vi "punto3_readfrom.vi"() -> ()   [LabVIEW 2024]
uses:
  <vilib>/express/express analysis/Spectral/Block/exnSpectralBlock spectral measurements peak poly.vi
  <vilib>/express/express analysis/Spectral/Block/exnSpectralBlock spectral measurements peak DDT.vi
  <vilib>/express/express analysis/Spectral/Block/exnSpectralBlock spectral measurements power poly.vi
  <vilib>/express/express analysis/Spectral/Block/exnSpectralBlock spectral measurements power DDT.vi
  <vilib>/express/express analysis/Spectral/XNode/ExpressSpectralMeasurementsBlockNode.xnode
panel:
  out "SINAD":dbl
  out "THD":dbl
  out "NOISE":dynamicdata(graph)
  out "SNR":dbl
  out "dt":dbl
  out "Y":dbl[](array[numeric])
  out "SIGNAL":dynamicdata(graph)
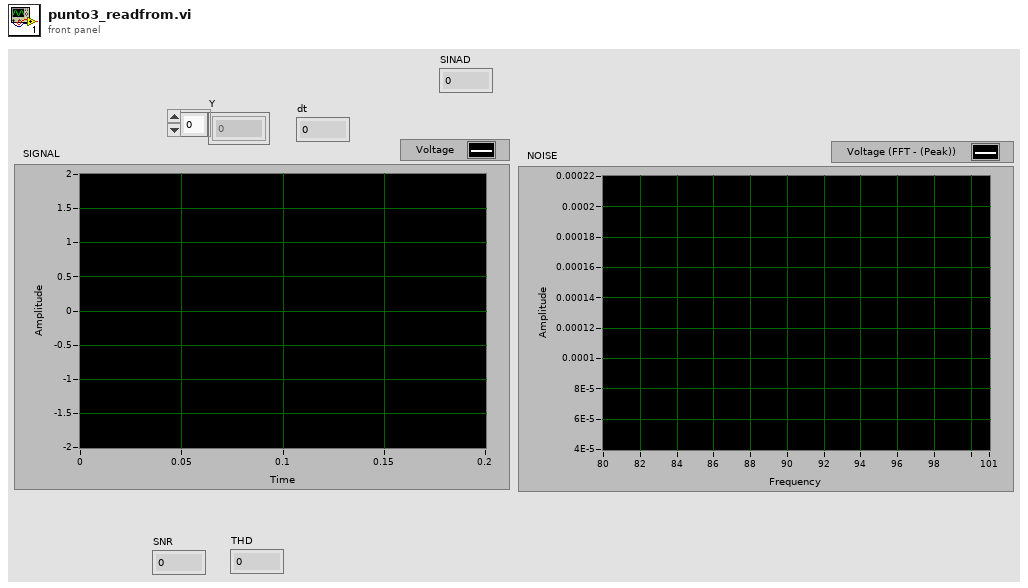
[diagram p1: front panel]
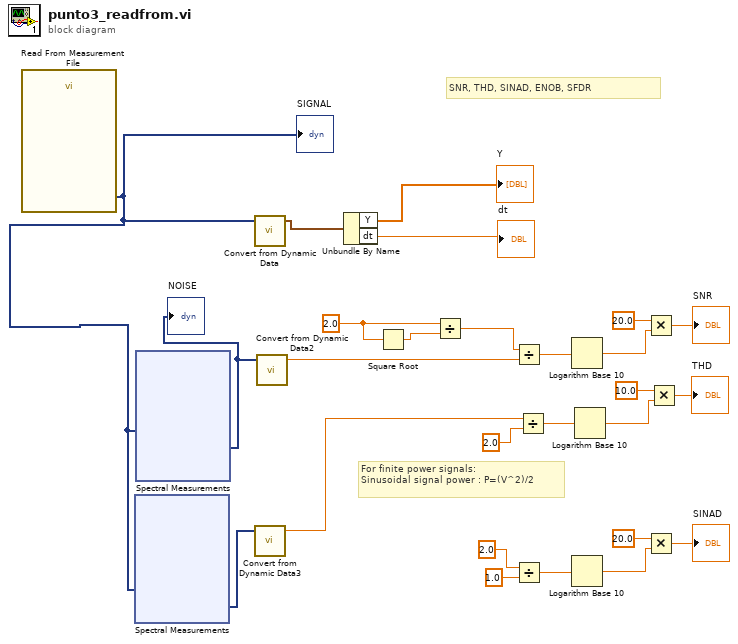
[diagram p0: block diagram]
diagram:
  w18 = 2.0 ("x")
  # "For finite power signals:\nSinusoidal signal power : P=(V^2)/2"
  # "SNR, THD, SINAD, ENOB, SFDR"
  n1 = call "Read From Measurement File"() -> ("Signals"=w1:dynamicdata)  [unwired: 6 in, 5 out]
  "SIGNAL" <- w1
  n2 = xnode "Spectral Measurements"("Signals"=w1) -> ("Power Spectrum"=w10:dynamicdata)  [unwired: 1 in, 1 out]
  n3 = xnode "Spectral Measurements"("Signals"=w1) -> ("FFT - (Peak)"=w16:dynamicdata)  [unwired: 1 in, 2 out]
  "NOISE" <- w16
  n4 = call "Convert from Dynamic Data"("Dynamic Data Type"=w1) -> ("Waveform"=w21:waveform(dbl))  [unwired: 3 in]
  n5 = call "Convert from Dynamic Data3"("Dynamic Data Type"=w10) -> ("Scalar"=w9:dbl)  [unwired: 3 in]
  n6 = call "Convert from Dynamic Data2"("Dynamic Data Type"=w16, "Channel"=w16) -> ("Scalar"=w15:dbl)  [unwired: 2 in]
  n7 = Unbundle By Name(w21) -> ("Y"=→"Y":dbl[], "dt"=→"dt":dbl)
  n8 = Square Root(x=w18) -> (sqrt(x)=w19:dbl)
  n9 = Divide(x=w18, y=w19) -> (x/y=w20:dbl)
  n10 = Divide(x=w20, y=w15) -> (x/y=w22:dbl)
  n11 = Divide(x=2.0, y=1.0) -> (x/y=w4:dbl)
  n12 = Divide(x=w9, y=2.0) -> (x/y=w11:dbl)
  n13 = Logarithm Base 10(1:w22) -> (0:w23:dbl)
  n14 = Logarithm Base 10(1:w4) -> (0:w6:dbl)
  n15 = Logarithm Base 10(1:w11) -> (0:w13:dbl)
  n16 = Multiply(x=20.0, y=w23) -> (x*y=→"SNR":dbl)
  n17 = Multiply(x=20.0, y=w6) -> (x*y=→"SINAD":dbl)
  n18 = Multiply(x=10.0, y=w13) -> (x*y=→"THD":dbl)
